vi "SettingParameters.vi"(8 "error in":errorcluster) -> (0 "error out":errorcluster, 3 "Parameters":T1={"hidden_layer_sizes"=[100.0], "activation"="relu", "solver"="adam", "alpha"=0.0001, "batch_size"={"batch_size_type"="auto", "batch_size_int"=32.0}, "learning_rate"="constant", "learning_rate_init"=0.001, "power_t"=0.5, "max_iter"=200.0, "shuffle"=TRUE, "random_state"=0.0, "tol"=0.0001, "verbose"=FALSE, "warm_start"=FALSE, "momentum"=0.9, "nesterovs_momentum"=TRUE, "early_stopping"=FALSE, "validation_fraction"=0.1, "beta_1"=0.999, "beta_2"=0.999, "epsilon"=1e-08, "n_iter_no_change"=10.0, "max_fun"=15000.0})   [LabVIEW 2020]
doc: "Set model parameters"
uses:
  Model/Supervised/MultiLayerPerceptron/MLPClassifier/Controls/mlp_classifier_params.ctl
panel:
  in  "Local Parameters":T1={"hidden_layer_sizes"=[100.0], "activation"="relu", "solver"="adam", "alpha"=0.0001, "batch_size"={"batch_size_type"="auto", "batch_size_int"=32.0}, "learning_rate"="constant", "learning_rate_init"=0.001, "power_t"=0.5, "max_iter"=200.0, "shuffle"=TRUE, "random_state"=0.0, "tol"=0.0001, "verbose"=FALSE, "warm_start"=FALSE, "momentum"=0.9, "nesterovs_momentum"=FALSE, "early_stopping"=FALSE, "validation_fraction"=0.1, "beta_1"=0.999, "beta_2"=0.999, "epsilon"=1e-08, "n_iter_no_change"=10.0, "max_fun"=15000.0}
  in  "Set":bool
  in  "R/W params":T1={"hidden_layer_sizes"=[100.0], "activation"="relu", "solver"="adam", "alpha"=0.0001, "batch_size"={"batch_size_type"="auto", "batch_size_int"=32.0}, "learning_rate"="constant", "learning_rate_init"=0.001, "power_t"=0.5, "max_iter"=200.0, "shuffle"=TRUE, "random_state"=0.0, "tol"=0.0001, "verbose"=FALSE, "warm_start"=FALSE, "momentum"=0.9, "nesterovs_momentum"=FALSE, "early_stopping"=FALSE, "validation_fraction"=0.1, "beta_1"=0.999, "beta_2"=0.999, "epsilon"=1e-08, "n_iter_no_change"=10.0, "max_fun"=15000.0}
  # "Parameters"
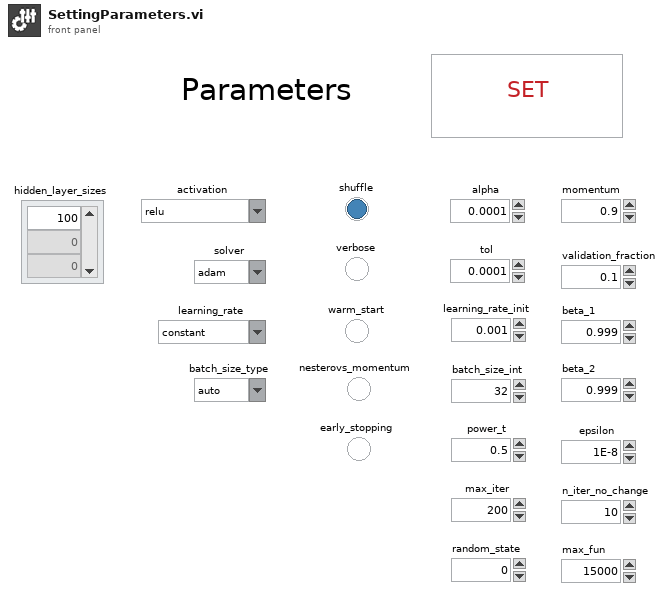
[diagram p1: front panel]
types:
  T1 = typedef "mlp_classifier_params.ctl" = cluster{"hidden_layer_sizes":dbl[], "activation":string, "solver":string, "alpha":dbl, "batch_size":cluster{"batch_size_type":string, "batch_size_int":dbl}, "learning_rate":string, "learning_rate_init":dbl, "power_t":dbl, "max_iter":dbl, "shuffle":bool, "random_state":dbl, "tol":dbl, "verbose":bool, "warm_start":bool, "momentum":dbl, "nesterovs_momentum":bool, "early_stopping":bool, "validation_fraction":dbl, "beta_1":dbl, "beta_2":dbl, "epsilon":dbl, "n_iter_no_change":dbl, "max_fun":dbl}
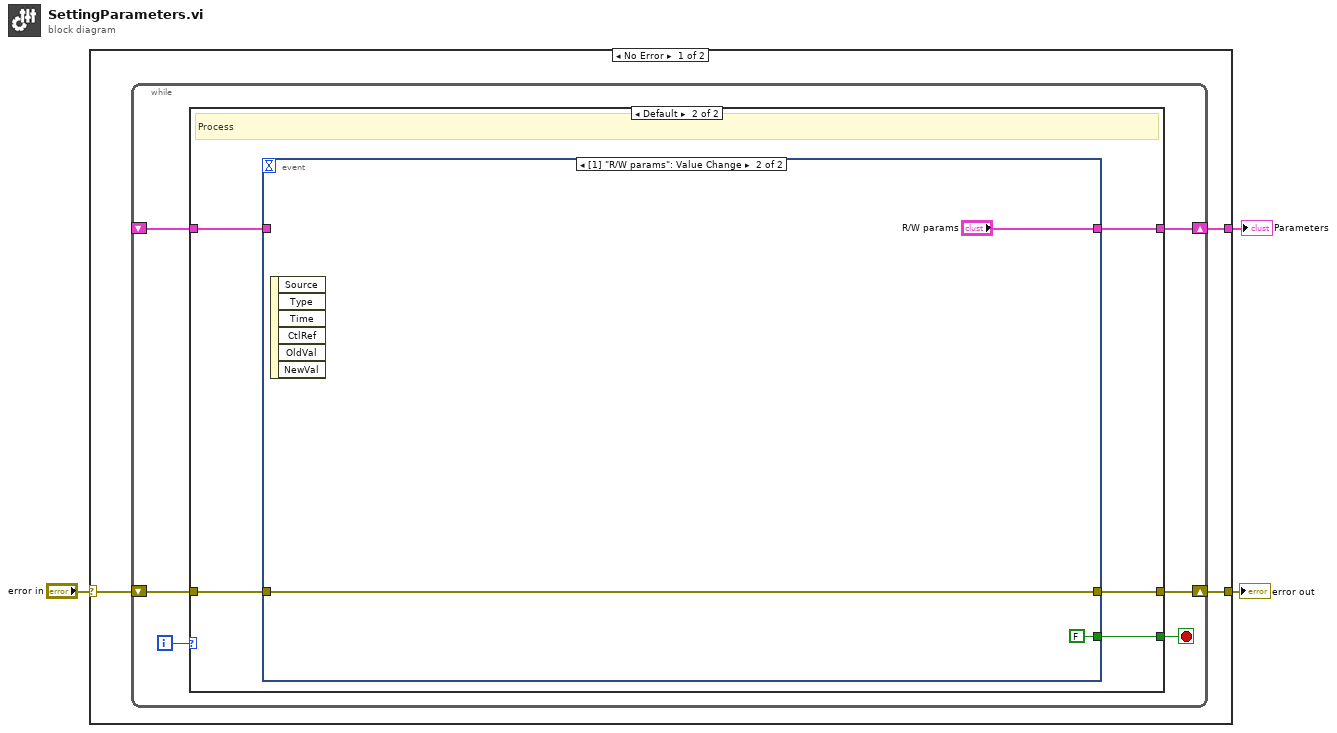
[diagram p0: block diagram]
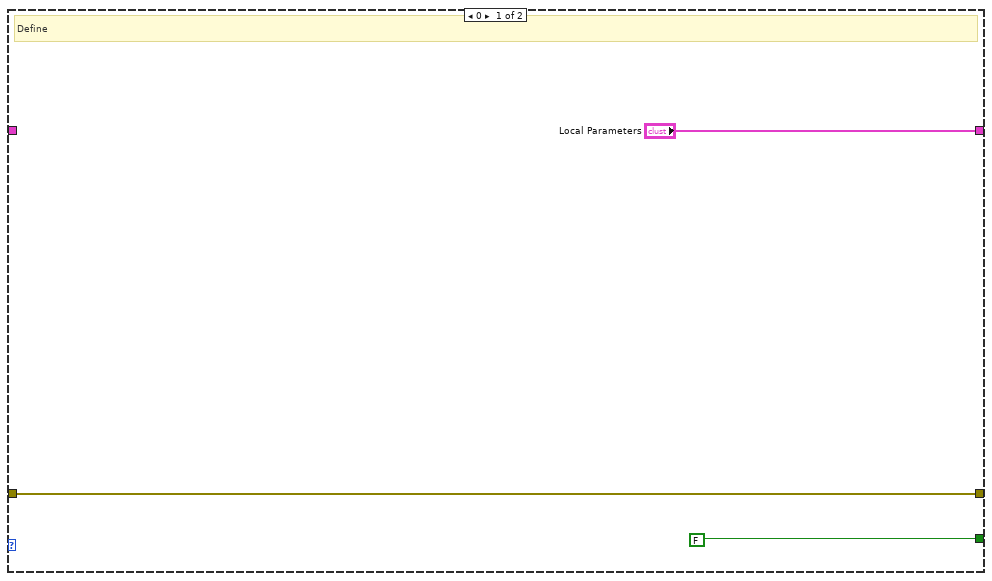
[diagram p2: hidden frame]
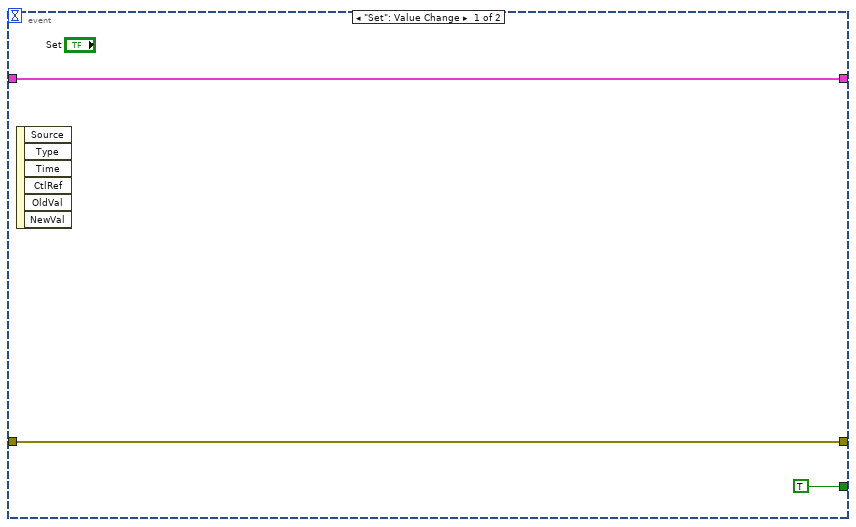
[diagram p3: hidden frame]
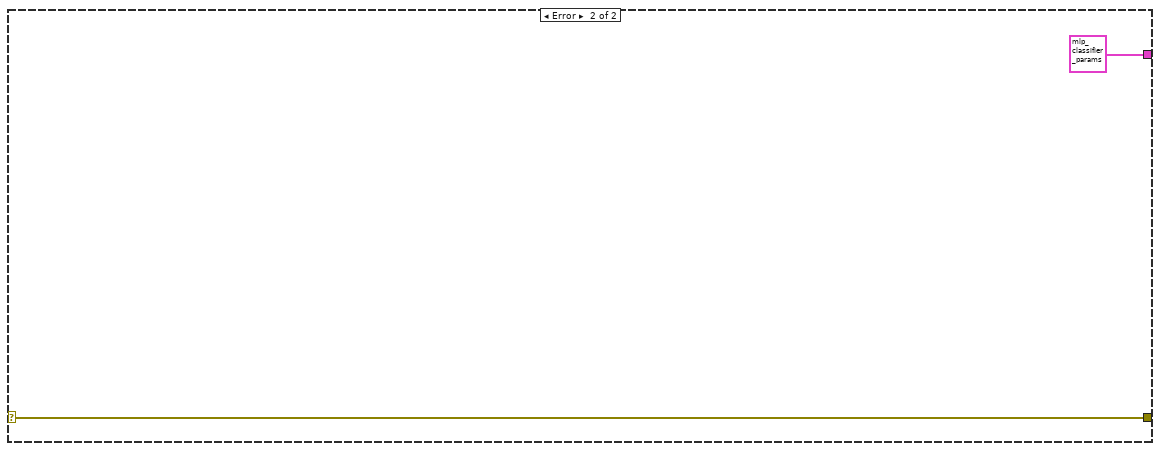
[diagram p4: hidden frame]
diagram:
  n1 = case shown="No Error" "error in" {
    selector: "error in" -> [w6 w28]
    tunnel: [w5 w28] -> w3
    tunnel: [w4 T1 {"hidden_layer_sizes"=[100.0], "activation"="relu", "solver"="adam", "alpha"=0.0001, "batch_size"={"batch_size_type"="auto", "batch_size_int"=32.0}, "learning_rate"="constant", "learning_rate_init"=0.001, "power_t"=0.5, "max_iter"=200.0, "shuffle"=TRUE, "random_state"=0.0, "tol"=0.0001, "verbose"=FALSE, "warm_start"=FALSE, "momentum"=0.9, "nesterovs_momentum"=TRUE, "early_stopping"=FALSE, "validation_fraction"=0.1, "beta_1"=0.999, "beta_2"=0.999, "epsilon"=1e-08, "n_iter_no_change"=10.0, "max_fun"=15000.0} ("R/W params")] -> w1
    frame No Error {
      n2 = while {
        shift-right: [w10] -> w5
        shift-left: w6 -> [w12]
        shift-right: [w9] -> w4
        shift-left: _ -> [w11]
        i -> [w7]
        stop <- w8 stop-if-true
        n3 = case shown="Default" w7 {
          tunnel: w12 -> [w15 w20]
          tunnel: w11 -> [_ w19]
          tunnel: [w15 w17] -> w10
          tunnel: ["Local Parameters" w18] -> w9
          tunnel: [FALSE w16] -> w8
          frame 0 {
            # "Define"
          }
          frame Default {
            # "Process"
            n4 = event shown="[1] \"R/W params\": Value Change" {
              selector: _ -> [_ _]
              dyn-events: _ -> [_ _]
              timeout: _ -> [_ _]
              tunnel: w20 -> [w23 w25]
              tunnel: [w23 w25] -> w17
              tunnel: w19 -> [w22 _]
              tunnel: [w22 "R/W params"] -> w18
              tunnel: [TRUE FALSE] -> w16
              event "Set": Value Change {
                n5 = event-data() -> ()  [unwired: 1 in, 6 out]
              }
              event Value Change {
                n6 = event-data() -> ()  [unwired: 1 in, 6 out]
              }
            }
          }
        }
      }
    }
    frame Error {
    }
  }
  "error out" <- w3
  "Parameters" <- w1
